vi "Finalize.vi"(8 "error in (no error)":errorcluster, 11 "BaseSpecPage in":refnum<class "BaseSpecPage.lvclass">) -> (0 "error out":errorcluster, 2 "MetaDataObj out":refnum<class "MetaDataObj.lvclass">, 3 "BaseSpecPage out":refnum<class "BaseSpecPage.lvclass">)   [LabVIEW 2016, in "BaseSpecPage.lvclass"]
uses:
  <resource>/dialog/NewProjectWizard/SpecPage/Base/BaseSpecPage.lvclass
  <resource>/dialog/NewProjectWizard/MetaDataObj/MetaDataObj.lvclass
  <resource>/dialog/NewProjectWizard/SpecPage/Base/BaseSpecPage.lvclass/BaseSpecPage.ctl
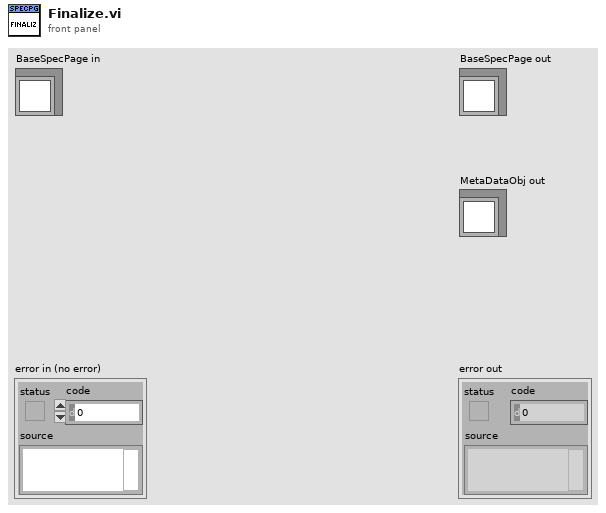
[diagram p1: front panel]
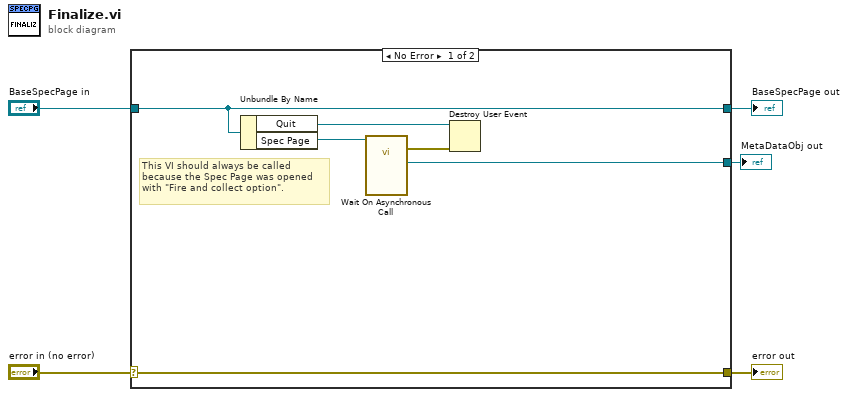
[diagram p0: block diagram]
diagram:
  n1 = case shown="No Error" "error in (no error)" {
    selector: "error in (no error)" -> [w6 w13]
    tunnel: [w6 w13] -> w4
    tunnel: [w11 w12] -> w2
    tunnel: "BaseSpecPage in" -> [w11 w12]
    tunnel: [w9 _] -> w1
    frame No Error {
      # "This VI should always be called\nbecause the Spec Page was opened\nwith \"Fire and collect option\"."
      n2 = Unbundle By Name(w11) -> ("Quit"=w7:refnum<user-event>, "Spec Page"=w10:refnum<vi>)
      n3 = call-by-ref "Wait On Asynchronous Call"(reference=w10) -> (error out=w8:errorcluster, "MetaDataObj out"=w9:refnum<class "MetaDataObj.lvclass">)  [unwired: 12 in, 1 out]
      n4 = Destroy User Event(user event=w7, error in=w8) -> ()  [unwired: 1 out]
    }
    frame Error {
    }
  }
  "error out" <- w4
  "BaseSpecPage out" <- w2
  "MetaDataObj out" <- w1
